vi "DrawJoystick.vi"(11 "Joystick":T2) -> (3 "DrawJoy":T1 {"Slide" scale=-1.0..1.0; "Trigger" scale=-1.0..1.0})   [LabVIEW 2012]
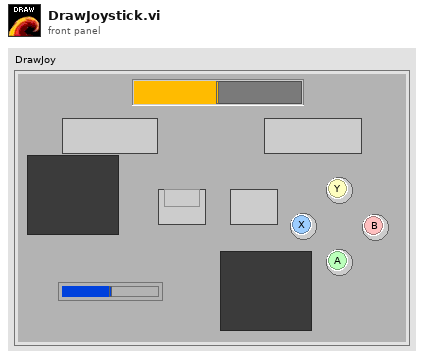
[diagram p1: front panel]
types:
  T1 = cluster{"Y":bool, "B":bool, "X":bool, "A":bool, "Left Bumper":bool, "Right Bumper":bool, "Joystick 2":cluster{"X":dbl, "Y":dbl}[], "Joystick 3":cluster{"X":dbl, "Y":dbl}[], "Back":bool, "Start":bool, "Trigger":dbl, "Slide":dbl, "Right Thumbstick":bool, "Left Thumbstick":bool}
  T2 = cluster{"Buttons":cluster{"A":bool, "B":bool, "X":bool, "Y":bool, "Left Bumper":bool, "Right Bumper":bool, "Back":bool, "Start":bool, "Left Thumbstick":bool, "Right Thumbstick":bool}, "Axes":cluster{"Left Stick X ":dbl, "Left Stick Y":dbl, "Triggers":dbl, "Right Stick X":dbl, "Right Stick Y":dbl, "D-Pad X":dbl}}
  T3 = cluster{"Y":bool, "B":bool, "X":bool, "A":bool, "Left Bumper":bool, "Right Bumper":bool, "Joystick 2":cluster{"X":dbl, "Y":dbl}[], "Joystick 3":cluster{"X":dbl, "Y":dbl}[], "Back":bool, "Start":bool, "Trigger":dbl, "Slide":dbl, "Left Thumbstick":bool, "Right Thumbstick":bool}
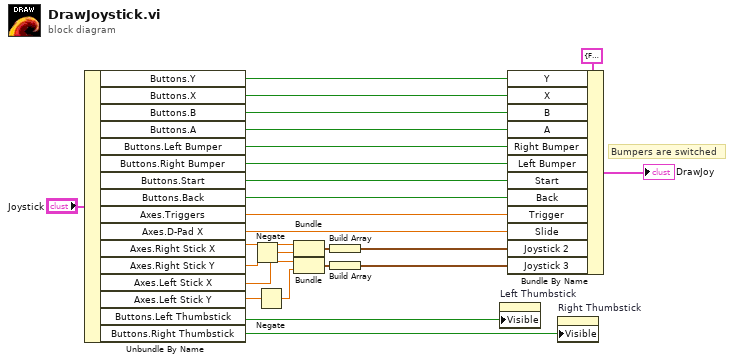
[diagram p0: block diagram]
diagram:
  # "Bumpers are switched"
  n1 = Unbundle By Name("Joystick") -> ("Buttons.Y"=w20:bool, "Buttons.X"=w19:bool, "Buttons.B"=w18:bool, "Buttons.A"=w17:bool, "Buttons.Left Bumper"=w16:bool, "Buttons.Right Bumper"=w15:bool, "Buttons.Start"=w14:bool, "Buttons.Back"=w13:bool, "Axes.Triggers"=w4:dbl, "Axes.D-Pad X"=w12:dbl, "Axes.Right Stick X"=w11:dbl, "Axes.Right Stick Y"=w10:dbl, "Axes.Left Stick X"=w23:dbl, "Axes.Left Stick Y"=w1:dbl, "Buttons.Left Thumbstick"=w5:bool, "Buttons.Right Thumbstick"=w6:bool)
  n2 = Negate(x=w10) -> (-x=w3:dbl)
  n3 = Negate(x=w1) -> (-x=w2:dbl)
  n4 = Bundle("Right Stick X"=w11, w3) -> (w24:cluster{"Right Stick X":dbl, dbl})  [unwired: 1 in]
  n5 = Bundle("Left Stick X"=w23, w2) -> (w25:cluster{"Left Stick X ":dbl, dbl})  [unwired: 1 in]
  n6 = Build Array(w24) -> (w9:cluster{"Right Stick X":dbl, dbl}[])
  n7 = Build Array(w25) -> (w8:cluster{"Left Stick X ":dbl, dbl}[])
  n8 = property on="Left Thumbstick" class="Bool (strict)"("Visible"=w5) -> ()  [unwired: 2 in, 2 out]
  n9 = Bundle By Name(cluster=T3 {"Y"=FALSE, "B"=FALSE, "X"=FALSE, "A"=FALSE, "Left Bumper"=FALSE, "Right Bumper"=FALSE, "Joystick 2"=[], "Joystick 3"=[], "Back"=FALSE, "Start"=FALSE, "Trigger"=0.0, "Slide"=0.0, "Left Thumbstick"=FALSE, "Right Thumbstick"=TRUE} ("DrawJoy"), "Y"=w20, "X"=w19, "B"=w18, "A"=w17, "Right Bumper"=w16, "Left Bumper"=w15, "Start"=w14, "Back"=w13, "Trigger"=w4, "Slide"=w12, "Joystick 2"=w9, "Joystick 3"=w8) -> (→"DrawJoy":T3)
  n10 = property on="Right Thumbstick" class="Bool (strict)"("Visible"=w6) -> ()  [unwired: 2 in, 2 out]
